vi "Write channel group.vi"(8 "error in (no error)":errorcluster, 10 "channel group":string, 11 "channel config object in":refnum<class "channel config object.lvclass">) -> (0 "error out":errorcluster, 3 "channel config object out":refnum<class "channel config object.lvclass">)   [LabVIEW 2013, in "channel config object.lvclass"]
uses:
  channel config object.lvclass
  channel config object.lvclass/channel config object.ctl
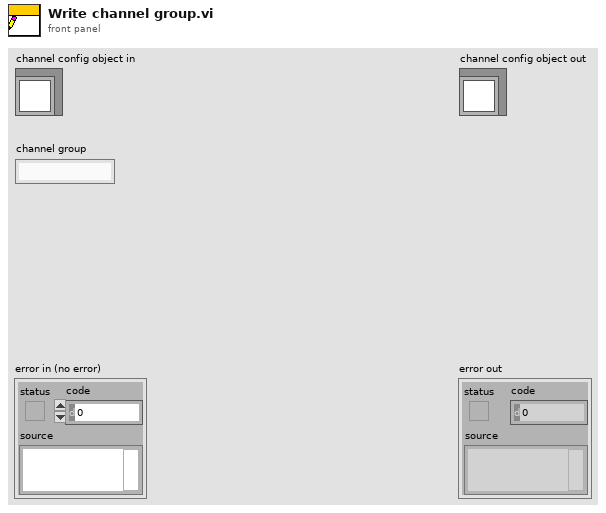
[diagram p1: front panel]
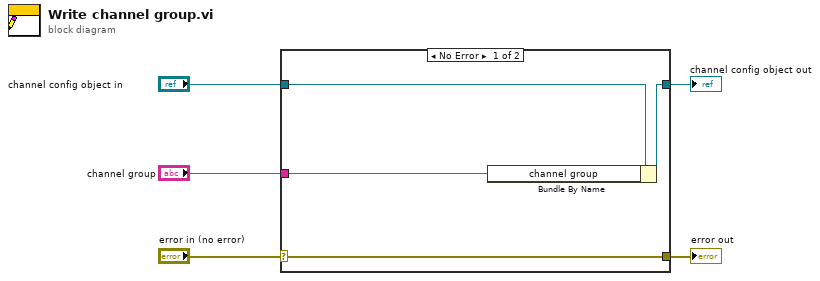
[diagram p0: block diagram]
diagram:
  n1 = case shown="No Error" "error in (no error)" {
    selector: "error in (no error)" -> [w9 w10]
    tunnel: [w9 w10] -> w4
    tunnel: [w7 w11] -> w2
    tunnel: "channel config object in" -> [w8 w11]
    tunnel: "channel group" -> [w6 _]
    frame No Error {
      n2 = Bundle By Name(cluster=w8, "channel group"=w6) -> (w7:refnum<class "channel config object.lvclass">)
    }
    frame Error {
    }
  }
  "error out" <- w4
  "channel config object out" <- w2
